vi "OFDM-SIM子载波解调.vi"(0 "输出符号":cdb[](array[numeric]) format="%#_6p") -> (1 "SIM输出":i32[](array[numeric]), 2 "去0后符号":cdb[](array[numeric]) format="%#_6p")   [LabVIEW 2018]
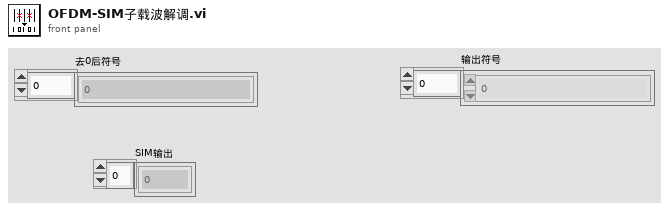
[diagram p1: front panel]
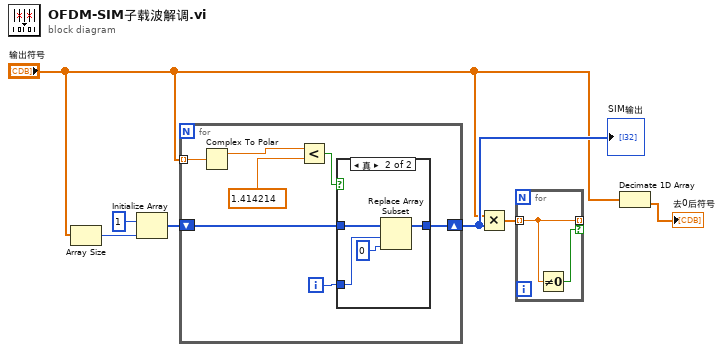
[diagram p0: block diagram]
diagram:
  n1 = Array Size(array="输出符号") -> (size(s)=w5:i32)
  n2 = Initialize Array(1, w5) -> (w6:i32[])
  n3 = for {
    tunnel: "输出符号" -> [w13] mode=indexing
    shift-right: [w9] -> w4
    shift-left: w6 -> [w11]
    i -> [w10]
    n4 = Complex To Polar(r * e^(i*theta)=w13) -> (r=w8:dbl)  [unwired: 1 out]
    n5 = Less?(x=w8, y=1.414214) -> (x < y?=w12:bool)
    n6 = case shown="真" w12 {
      tunnel: w11 -> [w15 w19]
      tunnel: w10 -> [_ w17]
      tunnel: [w15 w18] -> w9
      frame False {
      }
      frame True {
        n7 = Replace Array Subset(array=w19, new element=0, index=w17) -> (w18:i32[])
      }
    }
  }
  "SIM输出" <- w4
  n8 = Multiply(x="输出符号", y=w4) -> (x*y=w3:cdb[])
  n9 = for {
    tunnel: w3 -> [w20] mode=indexing
    tunnel: [w20] -> _ mode=indexing if=w21
    n10 = Not Equal To 0?(x=w20) -> (x != 0?=w21:bool)
  }
  n11 = Decimate 1D Array("输出符号") -> (→"去0后符号":cdb[])  [unwired: 1 out]
